vi "tsapp_get_bus_statistics.vi"(8 "错误输入（无错误）":errorcluster, 9 "TLIBCANBusStatistics":T1(ring), 10 "AIdxChn":T2(ring), 11 "ABusType":enum16{"APP_CAN", "APP_LIN"}(ring)) -> (0 "错误输出":errorcluster, 2 "AStat":dbl, 3 "tsapp_get_bus_statistics":i32)   [LabVIEW 2016]
uses:
  D:/Program Files (x86)/TOSUN/TSMaster/bin/Data/SDK/lib/x86/TSMaster.dll
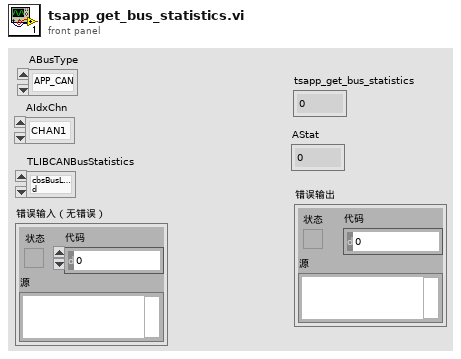
[diagram p1: front panel]
types:
  T1 = enum16{"cbsBusLoad", "cbsPeakLoad", "cbsFpsStdData", "cbsAllStdData", "cbsFpsExtData", "cbsAllExtData", "cbsFpsStdRemote", "cbsAllStdRemote", "cbsFpsExtRemote", "cbsAllExtRemote", "cbsFpsErrorFrame", "cbsAllErrorFrame"}
  T2 = enum16{"CHAN1", "CHAN2", "CHAN3", "CHAN4", "CHAN5", "CHAN6", "CHAN7", "CHAN8", "CHAN9", "CHAN10", "CHAN11", "CHAN12", "CHAN13", "CHAN14", "CHAN15", "CHAN16"}
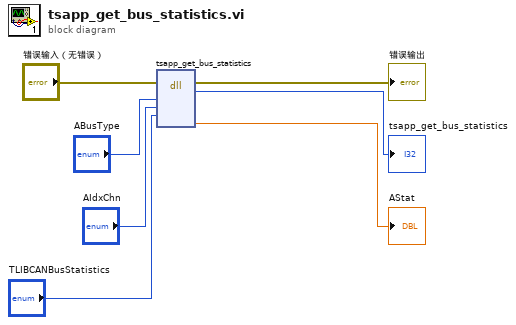
[diagram p0: block diagram]
diagram:
  n1 = dll-call lib="D:/Program Files (x86)/TOSUN/TSMaster/bin/Data/SDK/lib/x86/TSMaster.dll" fn="tsapp_get_bus_statistics"(error in="错误输入（无错误）", "ABusType"="ABusType", "AIdxChn"="AIdxChn", "TLIBCANBusStatistics"="TLIBCANBusStatistics") -> (error out=→"错误输出":errorcluster, "tsapp_get_bus_statistics"=→"tsapp_get_bus_statistics":i32, "AStat"=→"AStat":dbl)  [unwired: 6 in, 1 out]
